vi "ep_Check Max Order.vi"(8 "error in (no error)":errorcluster, 10 "maximum harmonic order":u16, 11 "samples per cycle":u16) -> (0 "error out":errorcluster)   [LabVIEW 2013, in "NI_EP_Power Measurement.lvlib"]
uses:
  <vilib>/addons/Electrical Power/Power Measurement/NI_EP_Power Measurement.lvlib
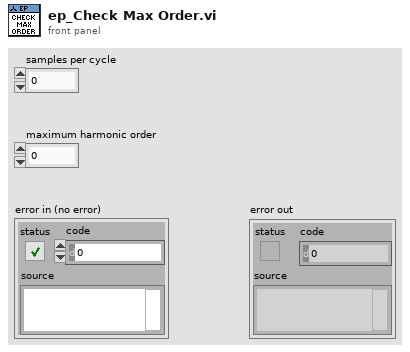
[diagram p1: front panel]
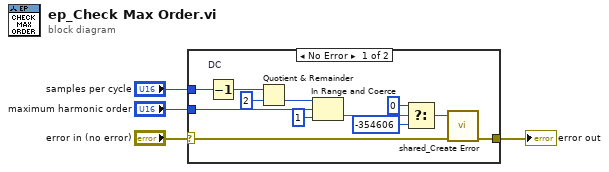
[diagram p0: block diagram]
diagram:
  n1 = case shown="No Error" "error in (no error)" {
    selector: "error in (no error)" -> [w9 w17]
    tunnel: "samples per cycle" -> [w12 _]
    tunnel: "maximum harmonic order" -> [w11 _]
    tunnel: [w8 w17] -> w1
    frame No Error {
      n2 = Decrement "DC"(x=w12) -> (x-1=w7:u16)
      n3 = Quotient & Remainder(x=w7, y=u16 2) -> (floor(x/y)=w5:u16)  [unwired: 1 out]
      n4 = In Range and Coerce(upper limit=w5, x=w11, lower limit=u16 1) -> (In Range?=w13:bool)  [unwired: 1 out]
      n5 = Select(t=0, s=w13, f=-354606) -> (s? t:f=w10:i32)
      n6 = call <vilib>:"shared_Create Error.vi"("error in (no error)"=w9, "error code (0)"=w10) -> ("error out"=w8:errorcluster)  [unwired: 9 in]
    }
    frame Error {
    }
  }
  "error out" <- w1
